vi "Insert Stop Message.vi"(8 "error in (no error)":errorcluster, 11 "Electrophysiology in":refnum<class "Electrophysiology.lvclass">) -> (0 "error out":errorcluster, 3 "Electrophysiology out":refnum<class "Electrophysiology.lvclass">)   [LabVIEW 2014, in "Electrophysiology.lvclass"]
uses:
  Electrophysiology.lvclass
  Database/EphysPrimary.ctl
  AcquistionObject/AcquistionObject.lvclass
panel:
  out "resulting string":string
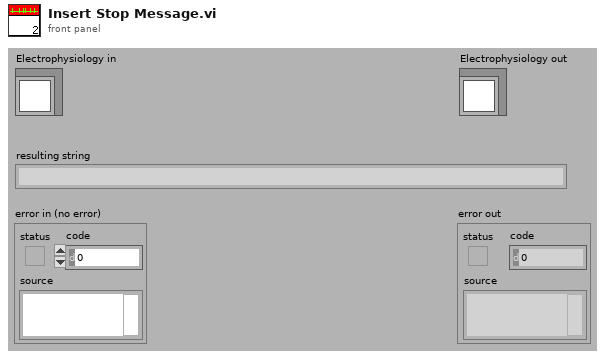
[diagram p1: front panel]
types:
  T1 = typedef "EphysPrimary.ctl" = cluster{"setup":u8, "subject_id":i32, "session_start_time":dbl, "ephys_start_time":dbl}
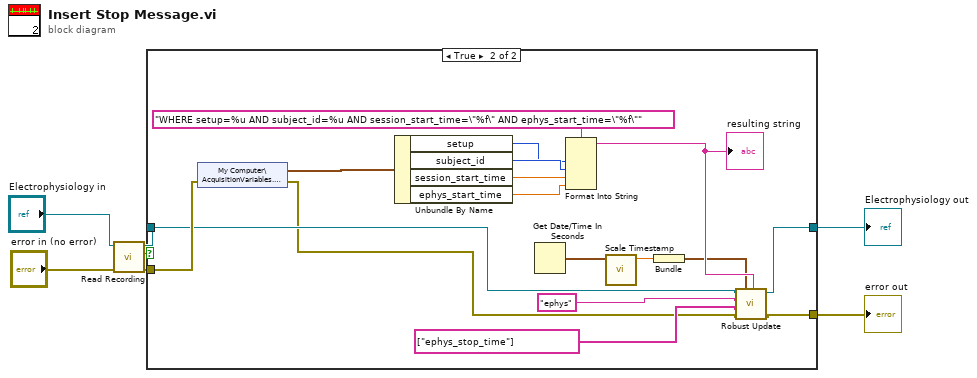
[diagram p0: block diagram]
diagram:
  n1 = call-dynamic "Read Recording.vi"("error in (no error)"="error in (no error)", "AcquireTraces in"="Electrophysiology in") -> ("error out"=w1:errorcluster, "Recording"=w5:bool, "AcquireTraces out"=w3:refnum<class "Electrophysiology.lvclass">)  [unwired: 7 in]
  n2 = case shown="True" w5 {
    tunnel: w1 -> [w8 w20]
    tunnel: [w8 w14] -> w7
    tunnel: [w9 w13] -> w6
    tunnel: w3 -> [w9 w12]
    frame False {
    }
    frame True {
      n3 = shared-variable "My Computer\\AcquisitionVariables.lvlib\\EphysPK"(error in=w20) -> (w25:T1, error out=w11:errorcluster)
      n4 = Unbundle By Name(w25) -> ("setup"=w10:u8, "subject_id"=w23:i32, "session_start_time"=w22:dbl, "ephys_start_time"=w19:dbl)
      n5 = Get Date/Time In Seconds() -> (seconds since 1Jan1904=w26:timestamp)
      n6 = Format Into String(format string="WHERE setup=%u AND subject_id=%u AND session_start_time=\"%f\" AND ephys_start_time=\"%f\"", w10, w23, w22, w19) -> (resulting string=w18:string)  [unwired: 2 in, 1 out]
      "resulting string" <- w18
      n7 = call "Scale Timestamp.vi"("Time Stamp"=w26) -> ("Scaled timestamp"=w21:dbl)  [unwired: 10 in]
      n8 = Bundle("Scaled timestamp"=w21) -> (w17:cluster{"Scaled timestamp":dbl})  [unwired: 1 in]
      n9 = call "Robust Update.vi"("condition"=w18, "data"=w17, "error in (no error)"=w11, "columns"=string[] ["ephys_stop_time"], "table"="ephys", "AcquistionObject.lvclass"=w12) -> ("error out"=w14:errorcluster, "AcquistionObject out"=w13:refnum<class "Electrophysiology.lvclass">)  [unwired: 4 in]
    }
  }
  "error out" <- w7
  "Electrophysiology out" <- w6
